vi "AOI List Globals.vi"() -> ()   [LabVIEW 2016]
panel:
  in  "Frame number":i32[](array[numeric])
  in  "Track number":u16[](array[numeric])
  in  "AOI List":u16[][](array[numeric])
  # "AOI list is x1 y1 x2 y2"
  # "-1 if in all frames"
  # "This file is part of Glimpse. \nCopyright 2014 Jeff Gelles, Brandeis University.    \n\nGlimpse is free software: you can redistribute it and/or modify it under the \nterms of the GNU General Public License as published by the Free Software \nFoundation, either version 3 of the License, or (at your option) any later \nversion.\n\nGlimpse is distributed in the hope that it will be useful, but WITHOUT ANY \nWARRANTY; without even the implied warranty of MERCHANTABILITY or FITNESS FOR \nA PARTICULAR PURPOSE.  See the GNU General Public License for more details.\n\nYou should have received a copy of the GNU General Public License\nalong with Glimpse.  If not, see <http://www.gnu.org/licenses/>."
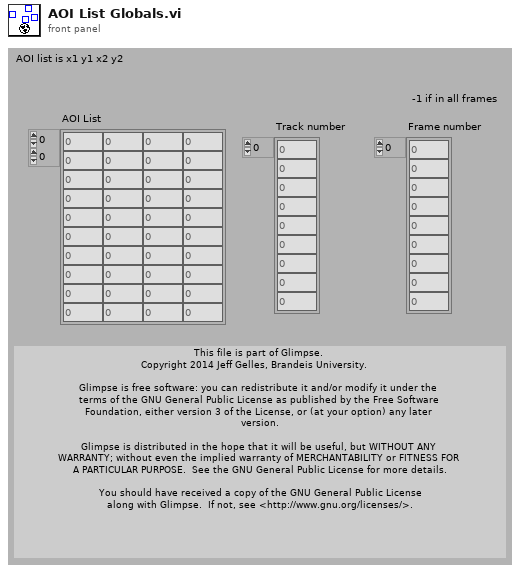
[diagram p1: front panel]
diagram:
